vi "Restarts by Flow Sandbox New (FPGA).vi"() -> ()   [LabVIEW 2019]
uses:
  Controls/SPI Channels.ctl
  <vilib>/Platform/TimedLoop/XDataNode/wakeup.ctl
  <vilib>/Platform/TimedLoop/XDataNode/XDNodeRunTimeDep.lvlib
  <vilib>/Platform/TimedLoop/XDataNode/nitl_modes.ctl
  <vilib>/Platform/TimedLoop/XDataNode/timing_clust.ctl
  <vilib>/Platform/TimedLoop/XDataNode/XDataNode.xnode
  <userlib>/_NI SPI IP/FPGA/Controllers/Public/Spi Master Inputs.ctl
  <vilib>/eio/EIONode/EIONode.xnode
  <vilib>/rvi/eio/common/nirviEmuTemplateMethod_errors.vi
  <vilib>/eio/EIOMethodNode/EIOMethodNode.xnode
  <vilib>/rvi/FXPMathLib/FxpMul/XNode/nifxpmath_Multiplier.xnode
  <vilib>/rvi/FXPMathLib/sim/FxpSim.dll
  <vilib>/rvi/FXPMathLib/FxpAdd/XNode/nifxpmath_Add.xnode
  <vilib>/rvi/DataTransferAndStorage/Container/XNode/niFpgaContainer.xnode
  <vilib>/rvi/interface/RandomDataEmulation/nirviRandomDataFpgaReadWriteTemplate.vi
  <userlib>/_NI SPI IP/FPGA/Controllers/Public/Transfer Settings.ctl
panel:
  in  "HighLimit":fxp<+/-,28,17>=13413.0 format="%#_17g"
  in  "LowLimit":fxp<+/-,28,17>=13238.0 format="%#_17g"
  in  "Trigger Span":i32=5
  in  "Reset Restarts":bool
  in  "Position":i32
  out "Current":fxp<+/-,28,17>
  out "Pressure":fxp<+/-,28,17>
  out "DetPres Starts":u32
  in  "AO0":fxp<+/-,20,5>
  in  "AI16-23 Data to Write":u64 format="%.0x"
  out "AI16-23":fxp<+/-,28,17>[](array[numeric])
  out "Read Data":u64 format="%.0x"
  in  "AI16-23 Settings":T1 {"Direction Change Bit" max=64 step=1; "Transfer Length (bits)" min=1 max=64 step=1}
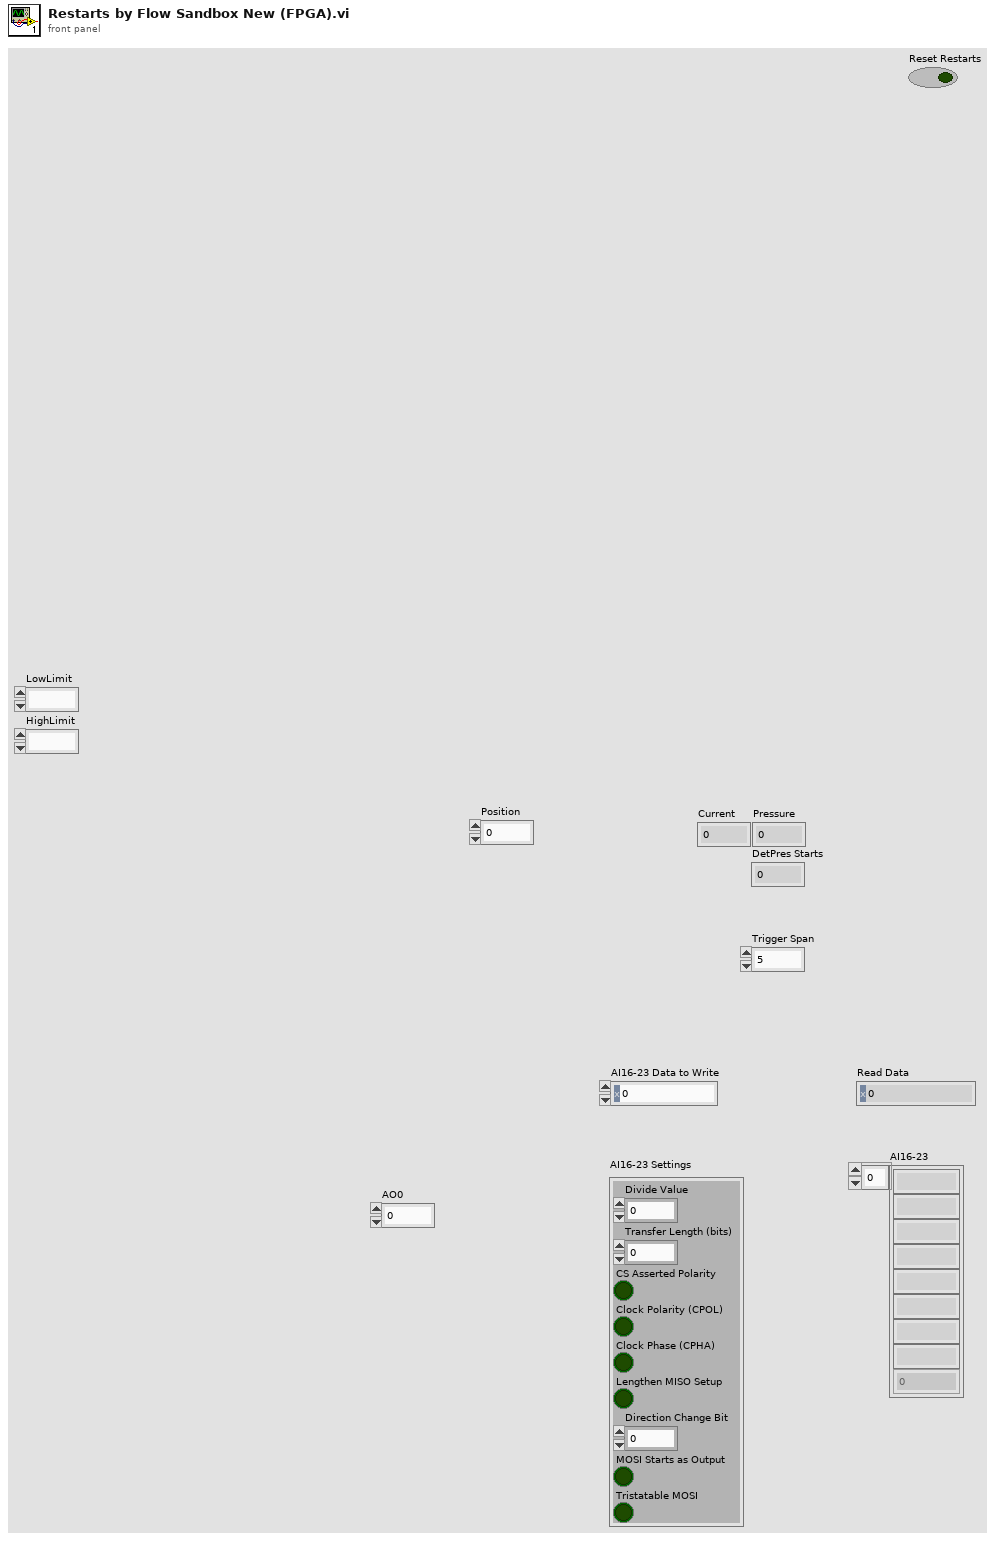
[diagram p1: front panel]
types:
  T1 = typedef "DIO SPI FPGA.lvlib/Transfer Settings.ctl" = cluster{"Divide Value":u8, "Transfer Length (bits)":u8, "CS Asserted Polarity":bool, "Clock Polarity (CPOL)":bool, "Clock Phase (CPHA)":bool, "Lengthen MISO Setup":bool, "Direction Change Bit":u8, "MOSI Starts as Output":bool, "Tristatable MOSI":bool}
  T2 = typedef "SPI Channels.ctl" = cluster{"CS":refnum<k21>, "CLK":refnum<k21>, "MOSI":refnum<k21>, "MISO":refnum<k21>}
  T3 = typedef "XDNodeRunTimeDep.lvlib/timing_clust.ctl" = cluster{"Expected End [f-1]":u64, "Actual End [f-1]":u64, "Finished Late? [f-1]":bool, "Expected End [i-1]":u64, "Actual End [i-1]":u64, "Finished Late? [i-1]":bool, "Expected Start [i]":u64, "Actual Start [i]":u64, "Expected Start [f]":u64, "Actual Start [f]":u64, "Source Name":string, "Structure Name":string, "Period":i64, "Deadline":i64, "Offset":i64, "Start":i64, "Priority":i32, "Timeout":i32, "Mode":T4, "Wakeup Reason":T5, "Error":errorcluster, "Source Type":string, "Secondary Source Type":string, "Global End Time":u64, "Global Start Time":u64, "Frame Duration":u64, "Iteration Duration":u64, "Assigned CPU":i32, "I/O Scan Engine Mode":u32}
  T4 = typedef "XDNodeRunTimeDep.lvlib/nitl_modes.ctl" = enum32{"No Change", "Process missed periods, maintain original phase", "Discard missed periods, maintain original phase", "Process missed periods, ignore original phase", "Discard missed periods, ignore original phase"}
  T5 = typedef "XDNodeRunTimeDep.lvlib/wakeup.ctl" = enum32{"Normal", "Aborted", "Asynchronous wakeup", "Timing source error", "Timed loop error", "Timeout"}
  T6 = typedef "DIO SPI FPGA.lvlib/Spi Master Inputs.ctl" = cluster{"MISO":bool}
  T7 = typedef "DIO SPI FPGA.lvlib/Spi Master Outputs.ctl" = cluster{"Chip Select":bool, "Clock":bool, "MOSI":bool, "MOSI OE":bool}
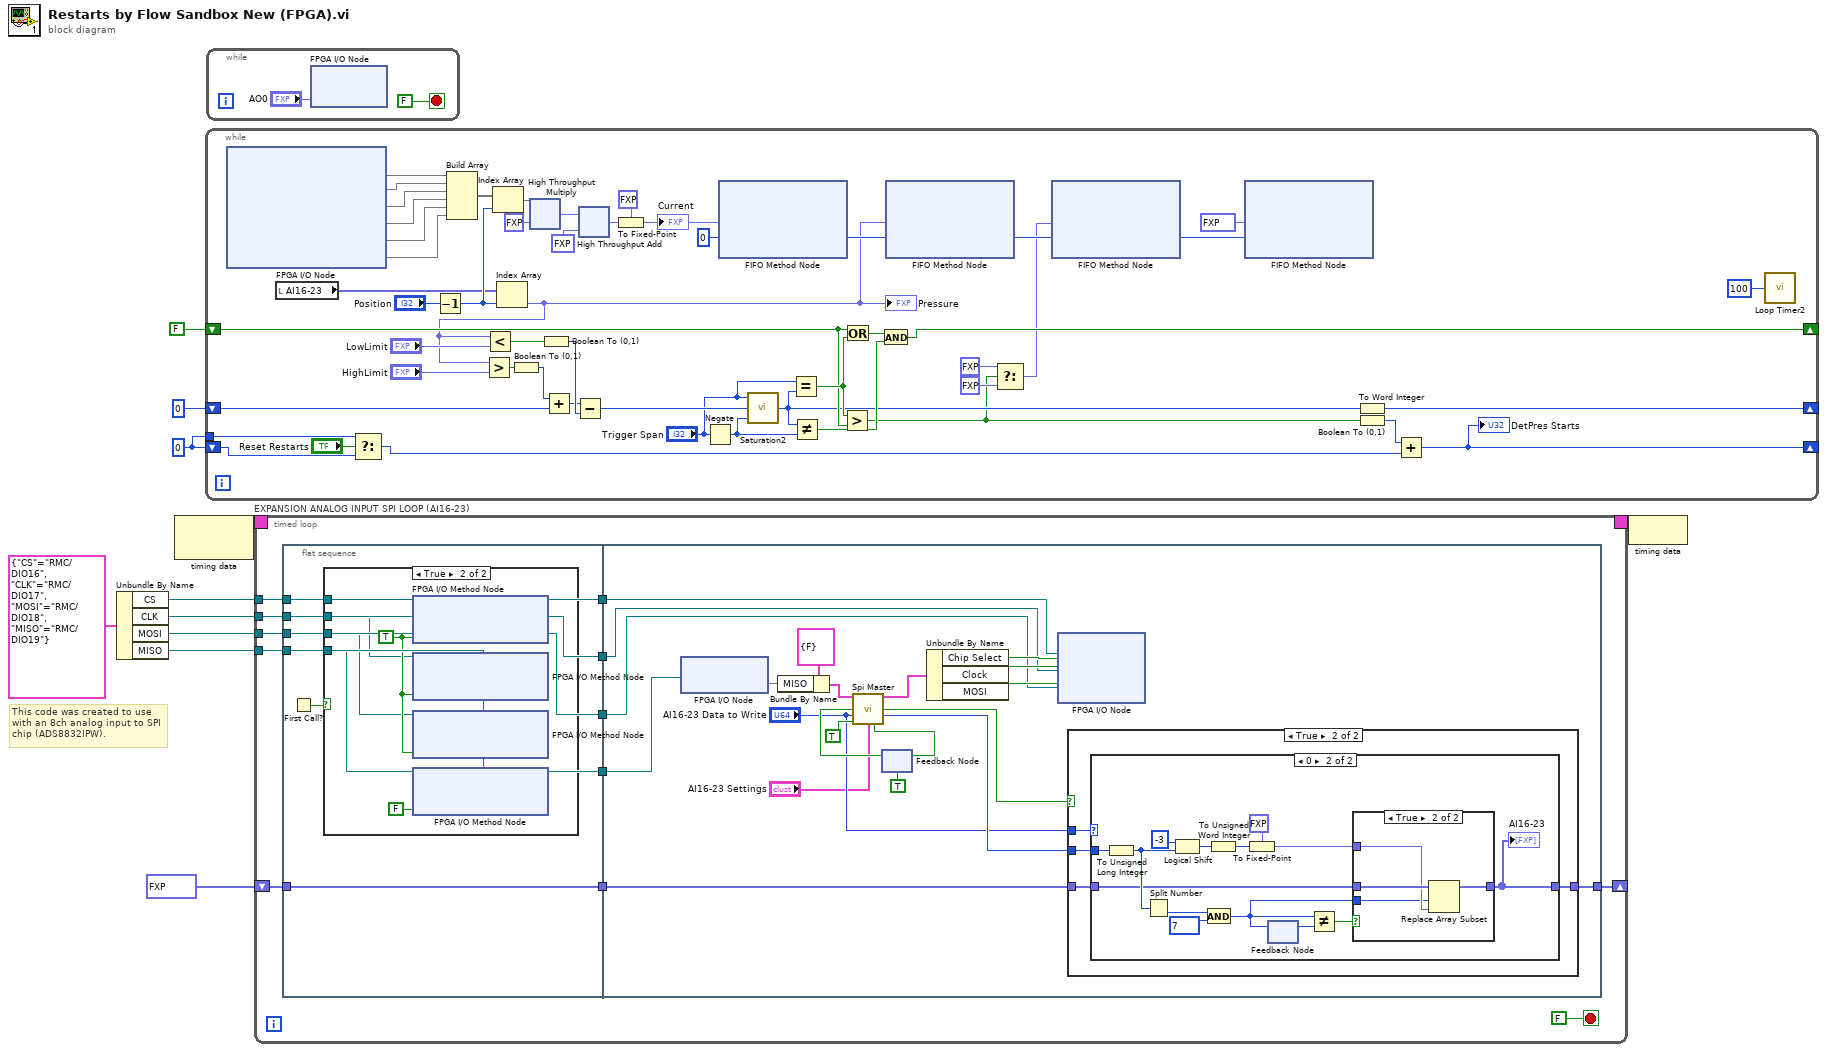
[diagram p0: block diagram]
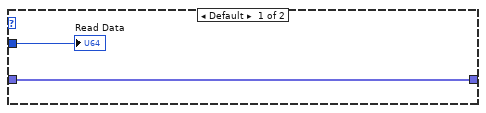
[diagram p4: hidden frame]
diagram:
  w1 = u32 0
  # "This code was created to use\nwith an 8ch analog input to SPI\nchip (ADS8832IPW)."
  n1 = Unbundle By Name(T2 {"CS"="RMC/DIO16", "CLK"="RMC/DIO17", "MOSI"="RMC/DIO18", "MISO"="RMC/DIO19"} ("SPI Channels")) -> ("CS"=w5:refnum<k21>, "CLK"=w6:refnum<k21>, "MOSI"=w7:refnum<k21>, "MISO"=w8:refnum<k21>)
  n2 = node-c288() -> (w11:T3)  [unwired: 1 in]
  n3 = while {
    shift-right: [w28] -> _
    shift-left: FALSE -> [w33]
    shift-right: [w29] -> _
    shift-left: i16 0 -> [w32]
    shift-right: [w30] -> _
    shift-left: w1 -> [w26]
    tunnel: w1 -> [w25]
    stop <- FALSE stop-if-true
    w18 = 0 ("Timeout")
    n4 = xnode "FPGA I/O Node"() -> ("Speed_Current_1 (AI0)"=w47, "Speed_Current_2 (AI1)"=w52, "Speed_Current_3 (AI2)"=w51, "Speed_Current_4 (AI3)"=w50, "Speed_Current_5 (AI4)"=w49, "Speed_Current_6 (AI5)"=w48)  [unwired: 6 in, 6 out]
    n5 = local read "AI16-23"() -> (w23:fxp<+/-,28,17>[])
    n6 = Select(t=w25, s="Reset Restarts", f=w26) -> (s? t:f=w27:u32)
    n7 = Decrement(x="Position") -> (x-1=w45:i32)
    n8 = Build Array(w47, w52, w51, w50, w49, w48) -> (w53:void[])
    n9 = Index Array(array=w53, index=w45) -> (element=w59)
    n10 = Index Array(array=w23, index=w45) -> (element=w17:fxp<+/-,28,17>)
    "Pressure" <- w17
    n11 = Greater?(x=w17, y="HighLimit") -> (0:w39:bool)
    n12 = Less?(x=w17, y="LowLimit") -> (x < y?=w38:bool)
    n13 = Boolean To (0,1)(Boolean=w39) -> (0, 1=w43:i16)
    n14 = xnode ("High Throughput Multiply")("x"=w59, "y"=fxp<+,5,5> 24.0 ("Current Scale")) -> ("x*y"=w56:fxp<+/-,29,10>)
    n15 = Boolean To (0,1)(Boolean=w38) -> (0, 1=w44:i16)
    n16 = Add(x=w43, y=w32) -> (x+y=w36:i16)
    n17 = Subtract(x=w36, y=w44) -> (x-y=w37:i16)
    n18 = xnode ("High Throughput Add")("x"=w56, "y"=fxp<+/-,7,7> -60.0 ("Current Offset")) -> ("x+y"=w58:fxp<+/-,30,11>)
    n19 = To Fixed-Point(fixed-point type=fxp<+/-,28,17> 0.0 ("out"), number=w58) -> (fixed-point=w19:fxp<+/-,28,17>)
    "Current" <- w19
    n20 = Negate(x="Trigger Span") -> (-x=w22:i32)
    n21 = xnode ("FIFO Method Node")("Element"=w19, "Timeout"=w18) -> ()  [unwired: 1 in, 2 out]
    n22 = call "Saturation2"("upper limit"="Trigger Span", "input"=w37, "lower limit"=w22) -> ("output"=w20:i32)  [unwired: 6 in]
    n23 = Equal?(x="Trigger Span", y=w20) -> (x = y?=w40:bool)
    n24 = Not Equal?(x=w20, y=w22) -> (x != y?=w42:bool)
    n25 = Greater?(x=w40, y=w33) -> (0:w14:bool)
    n26 = Or(x=w33, y=w40) -> (x .or. y?=w41:bool)
    n27 = And(x=w41, y=w42) -> (x .and. y?=w28:bool)
    n28 = xnode ("FIFO Method Node")("Element"=w17, "Timeout"=w18) -> ()  [unwired: 1 in, 2 out]
    n29 = Select(t=fxp<+/-,28,17> 1.0, s=w14, f=fxp<+/-,28,17> 0.0 ("Element")) -> (s? t:f=w13:fxp<+/-,28,17>)
    n30 = xnode ("FIFO Method Node")("Element"=w13, "Timeout"=w18) -> ()  [unwired: 1 in, 2 out]
    n31 = xnode ("FIFO Method Node")("Element"=fxp<+/-,28,17> -9999.0, "Timeout"=w18) -> ()  [unwired: 1 in, 2 out]
    n32 = To Word Integer(number=w20) -> (16bit integer=w29:i16)
    n33 = Boolean To (0,1)(Boolean=w14) -> (0, 1=w31:i16)
    n34 = Add(x=w31, y=w27) -> (x+y=w30:u32)
    "DetPres Starts" <- w30
    n35 = call "Loop Timer2"("Count(uSec)"=u32 100 ("Loop Timer (uSec)")) -> ()  [unwired: 1 out]
  }
  n36 = while {
    stop <- FALSE stop-if-true
    n37 = xnode "FPGA I/O Node"("AO0"="AO0") -> ()  [unwired: 2 in, 2 out]
  }
  n38 = timed-loop "EXPANSION ANALOG INPUT SPI LOOP (AI16-23)" {
    timing: w11 -> [_]
    timing-out: [_] -> w10
    shift-right: [w72] -> _
    shift-left: fxp<+/-,28,17>[] [0.0, 0.0, 0.0, 0.0, 0.0, 0.0, 0.0, 0.0] -> [w73]
    tunnel: w5 -> [w71]
    tunnel: w6 -> [w70]
    tunnel: w7 -> [w69]
    tunnel: w8 -> [w68]
    stop <- FALSE stop-if-true
    n39 = flat-sequence {
      tunnel: [w80] -> w74
      tunnel: w73 -> [w80]
      tunnel: w71 -> [w79]
      tunnel: w70 -> [w78]
      tunnel: w69 -> [w77]
      tunnel: w68 -> [w76]
      tunnel: [w79] -> w67
      tunnel: [w78] -> w66
      tunnel: [w77] -> w65
      tunnel: [w76] -> w64
      tunnel: w74 -> [w94]
      tunnel: [w93] -> w72
      tunnel: w67 -> [w92]
      tunnel: w66 -> [w91]
      tunnel: w65 -> [w90]
      tunnel: w64 -> [w89]
      frame #0 {
        n40 = First Call?() -> (First Call?: T/F=w81:bool)
        n41 = case shown="True" w81 {
          tunnel: w79 -> [_ w85]
          tunnel: w78 -> [_ w84]
          tunnel: w77 -> [_ w83]
          tunnel: w76 -> [_ w82]
          frame False {
          }
          frame True {
            w87 = TRUE ("Enable")
            n42 = xnode "FPGA I/O Method Node"("FPGA I/O In"=w85, "Enable"=w87) -> ()  [unwired: 1 out]
            n43 = xnode "FPGA I/O Method Node"("FPGA I/O In"=w84, "Enable"=w87) -> ()  [unwired: 1 out]
            n44 = xnode "FPGA I/O Method Node"("FPGA I/O In"=w83, "Enable"=w87) -> ()  [unwired: 1 out]
            n45 = xnode "FPGA I/O Method Node"("FPGA I/O In"=w82, "Enable"=FALSE) -> ()  [unwired: 1 out]
          }
        }
      }
      frame #1 {
        n46 = xnode "FPGA I/O Node"("FPGA I/O In"=w89) -> ("I/O Item"=w102)  [unwired: 1 out]
        n47 = Bundle By Name(cluster=T6 {"MISO"=FALSE} ("spi input"), "MISO"=w102) -> (w103:T6)
        n48 = feedback #1(TRUE ("read data valid")) -> (w99:bool)
        n49 = call <userlib>:"Spi Master.vi"("spi input"=w103, "start strobe"=w99, "data to write"="AI16-23 Data to Write", "MOSI output enable done"=TRUE, "spi transfer settings"="AI16-23 Settings") -> ("spi output"=w108:T7, "read data valid"=w95:bool, "read data"=w100:u64, "ready for input"=w96:bool)  [unwired: 7 in]
        n50 = feedback-in #1(w96) -> ()
        n51 = Unbundle By Name(w108) -> ("Chip Select"=w107:bool, "Clock"=w106:bool, "MOSI"=w105:bool)
        n52 = xnode "FPGA I/O Node"("I/O Item"=w107, "FPGA I/O In"=w92, "I/O Item"=w106, "FPGA I/O In"=w91, "I/O Item"=w105, "FPGA I/O In"=w90) -> ()  [unwired: 3 out]
        n53 = case shown="True" w95 {
          tunnel: w100 -> [_ w113]
          tunnel: "AI16-23 Data to Write" -> [_ w112]
          tunnel: w94 -> [w109 w111]
          tunnel: [w109 w110] -> w93
          frame False {
          }
          frame True {
            n54 = case shown="0" w112 {
              tunnel: w113 -> [w115 w129]
              tunnel: w111 -> [w114 w122]
              tunnel: [w114 w121] -> w110
              frame Default {
                "Read Data" <- w115
              }
              frame 0 {
                n55 = To Unsigned Long Integer(number=w129) -> (unsigned 32bit integer=w123:u32)
                n56 = Split Number(x=w123) -> (lo(x)=w127:u16)  [unwired: 1 out]
                n57 = Logical Shift(y=i16 -3, x=w123) -> (x << y=w124:u32)
                n58 = And(x=w127, y=u16 7) -> (x .and. y?=w119:u16)
                n59 = To Unsigned Word Integer(number=w124) -> (unsigned 16bit integer=w117:u16)
                n60 = To Fixed-Point(fixed-point type=fxp<+/-,28,17> 0.0 ("AI0"), number=w117) -> (fixed-point=w116:fxp<+/-,28,17>)
                n61 = feedback #2() -> (w128:u16)  [unwired: 1 in]
                n62 = feedback-in #2(w119) -> ()
                n63 = Not Equal?(x=w119, y=w128) -> (x != y?=w120:bool)
                n64 = case shown="True" w120 {
                  tunnel: w122 -> [w130 w134]
                  tunnel: [w130 w133] -> w121
                  tunnel: w119 -> [_ w131]
                  tunnel: w116 -> [_ w132]
                  frame False {
                  }
                  frame True {
                    n65 = Replace Array Subset(array=w134, new element=w132, index=w131) -> (w133:fxp<+/-,28,17>[])
                  }
                }
                "AI16-23" <- w121
              }
            }
          }
        }
      }
    }
  }
  n66 = node-c288(w10) -> ()
